vi "MotorControl.vi"   [LabVIEW 2017]
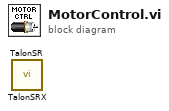
[diagram p0: block diagram]
diagram:
  n1 = call "TalonSRX.vi"() -> ()  [unwired: 3 in]
  n2 = call "TalonSR.vi"() -> ()  [unwired: 3 in]
